vi "test Prevent Overscroll.vi"(8 "error in (no error)":errorcluster, 11 "TestCase in":refnum<class "UI Common Unit Tests.lvclass">) -> (0 "error out":errorcluster, 3 "TestCase out":refnum<class "UI Common Unit Tests.lvclass">)   [LabVIEW 2017, in "UI Common Unit Tests.lvclass"]
uses:
  UI Common Unit Tests.lvclass
  Array Row.ctl
  <vilib>/addons/_JKI Toolkits/VI Tester/TestCase.llb/TestCase.lvclass
  UI Common.lvlib
  C:/Program Files (x86)/National Instruments/LabVIEW 2017/vi.lib/addons/_JKI Toolkits/VI Tester/TestCase.llb/TestCase.lvclass
panel:
  in  "Array":T1[](array[typedef])
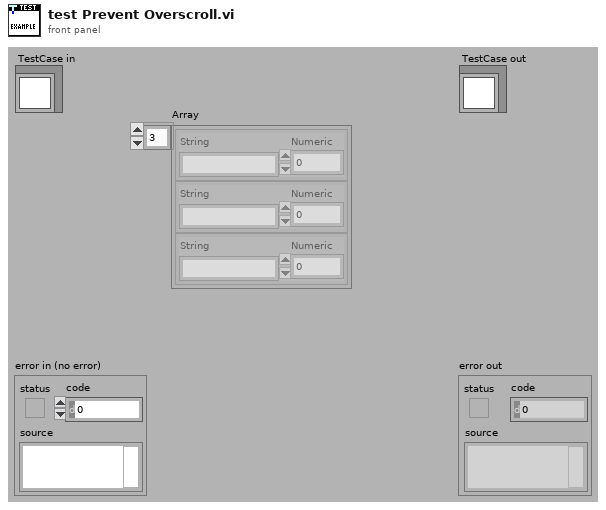
[diagram p1: front panel]
types:
  T1 = typedef "UI Common Unit Tests.lvclass/Array Row.ctl" = cluster{"String":string, "Numeric":dbl}
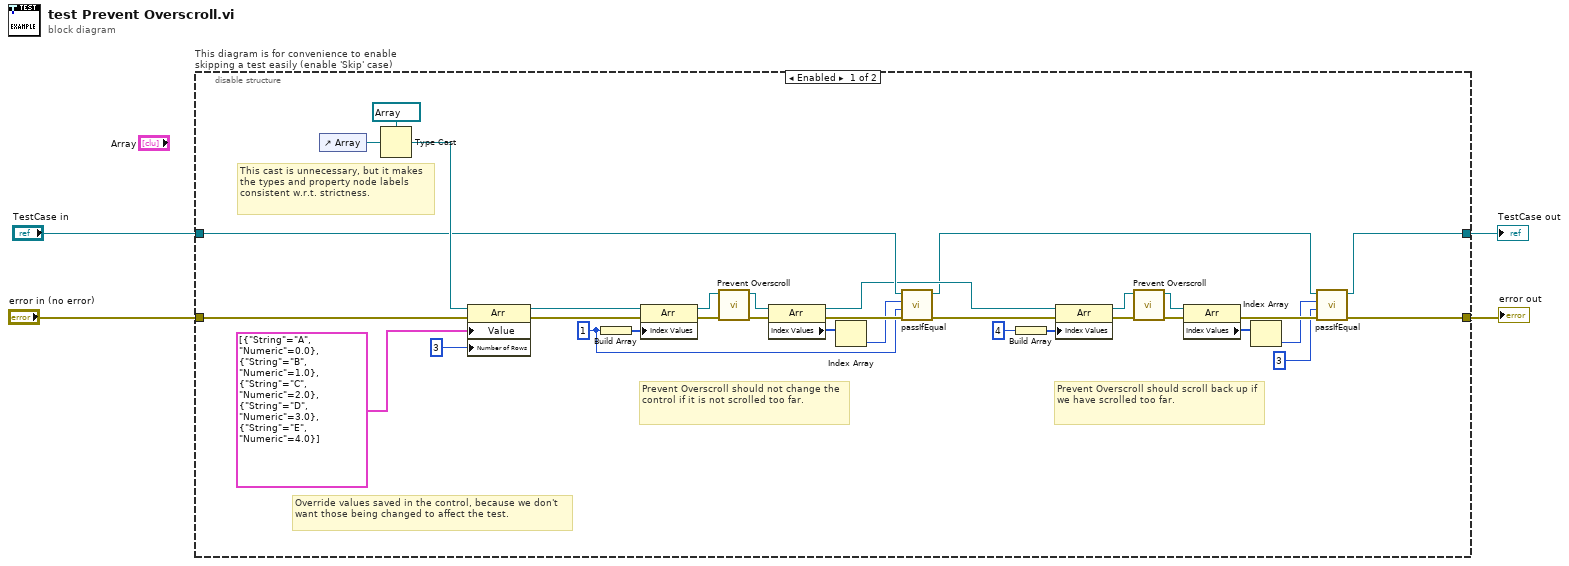
[diagram p0: block diagram]
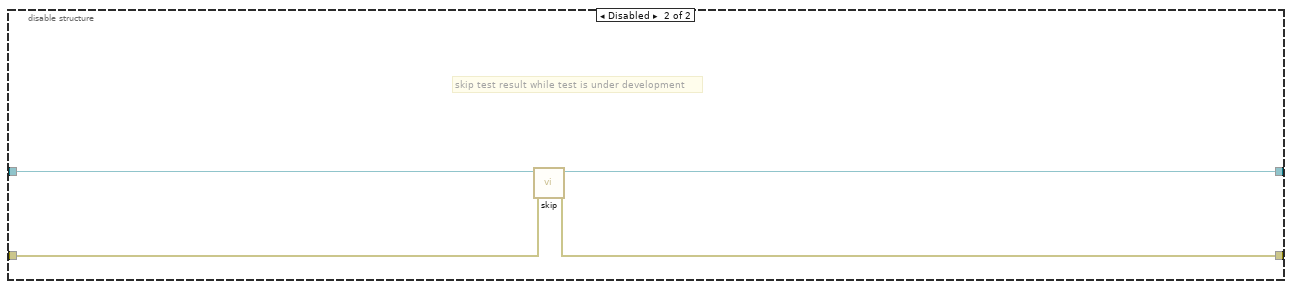
[diagram p2: hidden frame]
diagram:
  n1 = disable-structure "This diagram is for convenience to enable skipping a test easily (enable 'Skip' case)" shown="Enabled" {
    disable-tunnel: "TestCase in" -> [w23 w41]
    disable-tunnel: [w5 w39] -> w1
    disable-tunnel: [w7 w40] -> w3
    disable-tunnel: "error in (no error)" -> [w37 w38]
    frame Enabled {
      w8 = u32 1 ("Number of Rows")
      # "This cast is unnecessary, but it makes the types and property node labels consistent w.r.t. strictness."
      # "Prevent Overscroll should scroll back up if we have scrolled too far."
      # "Prevent Overscroll should not change the control if it is not scrolled too far."
      # "Override values saved in the control, because we don't want those being changed to affect the test."
      n2 = control-ref of="Array"() -> (w27:refnum<vi>)
      n3 = Type Cast(type=refnum<vi> refnum ("Array Refnum"), x=w27) -> (*(type *) &x=w25:refnum<vi>)
      n4 = property class="Arr"(reference=w25, error in=w37, "Value"=T1[] [{"String"="A", "Numeric"=0.0}, {"String"="B", "Numeric"=1.0}, {"String"="C", "Numeric"=2.0}, {"String"="D", "Numeric"=3.0}, {"String"="E", "Numeric"=4.0}], "Number of Rows"=u32 3) -> (reference out=w32:refnum<vi>, error out=w34:errorcluster)
      n5 = Build Array(w8) -> (w33:u32[])
      n6 = property class="Arr"(reference=w32, error in=w34, "Index Values"=w33) -> (reference out=w31:refnum<vi>, error out=w30:errorcluster)
      n7 = call "Prevent Overscroll.vi"("error in (no error)"=w30, "Array Refnum"=w31) -> ("error out"=w28:errorcluster, "Array Refnum"=w29:refnum<vi>)  [unwired: 8 in]
      n8 = property class="Arr"(reference=w29, error in=w28) -> (reference out=w9:refnum<vi>, error out=w24:errorcluster, "Index Values"=w22:u32[])
      n9 = Index Array(array=w22) -> (element=w21:u32)  [unwired: 1 in]
      n10 = call-dynamic "passIfEqual.vi"("error in (no error)"=w24, "y"=w8, "x"=w21, "TestCase in"=w23) -> ("error out"=w10:errorcluster, "TestCase out"=w6:refnum<class "UI Common Unit Tests.lvclass">)  [unwired: 6 in]
      n11 = Build Array(u32 4 ("Number of Rows")) -> (w20:u32[])
      n12 = property class="Arr"(reference=w9, error in=w10, "Index Values"=w20) -> (reference out=w18:refnum<vi>, error out=w17:errorcluster)
      n13 = call "Prevent Overscroll.vi"("error in (no error)"=w17, "Array Refnum"=w18) -> ("error out"=w15:errorcluster, "Array Refnum"=w16:refnum<vi>)  [unwired: 8 in]
      n14 = property class="Arr"(reference=w16, error in=w15) -> (error out=w14:errorcluster, "Index Values"=w13:u32[])  [unwired: 1 out]
      n15 = Index Array(array=w13) -> (element=w12:u32)  [unwired: 1 in]
      n16 = call-dynamic "passIfEqual.vi"("error in (no error)"=w14, "y"=u32 3 ("element"), "x"=w12, "TestCase in"=w6) -> ("error out"=w7:errorcluster, "TestCase out"=w5:refnum<class "UI Common Unit Tests.lvclass">)  [unwired: 6 in]
    }
    frame Disabled {
      # "skip test result while test is under development"
      n17 = call <vilib>:"skip.vi"("error in (no error)"=w38, "TestCase in"=w41) -> ("error out"=w40:errorcluster, "TestCase out"=w39:refnum<class "UI Common Unit Tests.lvclass">)  [unwired: 8 in]
    }
  }
  "error out" <- w3
  "TestCase out" <- w1
